vi "Flowmeter - revA.vi"() -> ()   [LabVIEW 2018]
doc: "This example demonstrates how to continuously perform period, frequency, pulse width, or two edge separation measurement types.\n\nThis example uses implicit timing, which means that a sample is acquired for every period of your input signal.\n\nFor instructions on how to connect your signals to the DAQ device, refer to your device documentation."
uses:
  <vilib>/Utility/error.llb/DialogType.ctl
  <vilib>/DAQmx/read.llb/DAQmx Read (Counter DBL 1Chan 1Samp).vi
  <vilib>/DAQmx/create/channels.llb/DAQmx Create Channel (CI-Frequency).vi
  <vilib>/DAQmx/configure/timing.llb/DAQmx Timing (Implicit).vi
  <vilib>/DAQmx/miscellaneous.llb/DAQmx Fill In Error Info.vi
  <resource>/objmgr/daqmx.rc
panel:
  out "K-Factor":dbl
  in  "K-Factor":dbl[](array[numeric])
  in  "Range":dbl[](array[numeric])
  out "GPM":dbl
  in  "counter":tag
  in  "CI.Freq.Term":tag
  out "Frequency":dbl
  in  "Stop":bool
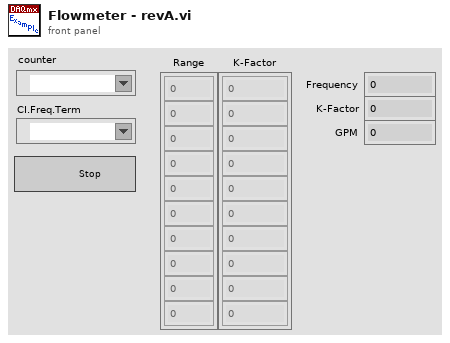
[diagram p1: front panel]
types:
  T1 = typedef "DialogType.ctl" = u16
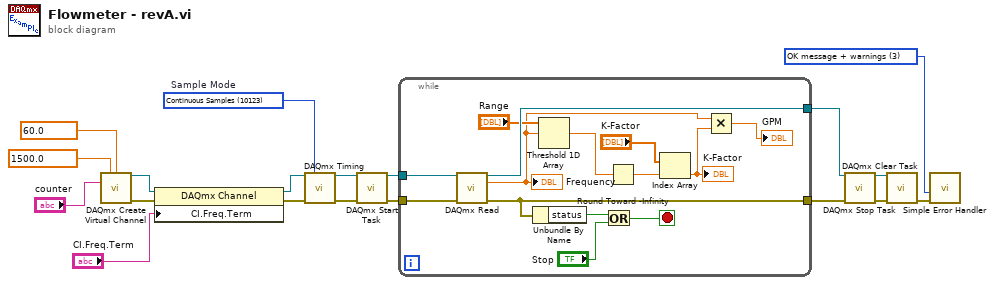
[diagram p0: block diagram]
diagram:
  w7 = T1 3 items=["no dialog", "OK message", "continue or stop message", "OK message + warnings", "continue/stop + warnings"] ("type of dialog (OK msg:1)")
  w19 = 10123 items=["Finite Samples"=10178, "Continuous Samples"=10123, "Hardware Timed Single Point"=12522]  # Sample Mode
  n1 = call-poly <vilib>:"DAQmx Create Virtual Channel.vi"("maximum value"=1500.0 ("Max Frequency"), "minimum value"=60.0 ("Min Frequency"), "counter"="counter") -> ("task out"=w6:refnum<k21>, "error out"=w5:errorcluster)  [unwired: 11 in]
  n2 = property class="DAQmx Channel"(reference=w6, error in=w5, "CI.Freq.Term"="CI.Freq.Term") -> (reference out=w17:refnum<k21>, error out=w18:errorcluster)
  n3 = call-poly <vilib>:"DAQmx Timing.vi"("task/channels in"=w17, "sample mode"=w19, "error in"=w18) -> ("task out"=w13:refnum<k21>, "error out"=w12:errorcluster)  [unwired: 11 in]
  n4 = call <vilib>:"DAQmx Start Task.vi"("task/channels in"=w13, "error in"=w12) -> ("task out"=w16:refnum<k21>, "error out"=w15:errorcluster)  [unwired: 12 in]
  n5 = while {
    tunnel: w16 -> [w33]
    tunnel: w15 -> [w32]
    tunnel: [w29] -> w8
    tunnel: [w30] -> w9
    stop <- w31 stop-if-true
    n6 = call-poly <vilib>:"DAQmx Read.vi"("task/channels in"=w33, "error in"=w32) -> ("task out"=w30:refnum<k21>, "data"=w20:dbl, "error out"=w29:errorcluster)  [unwired: 11 in]
    "Frequency" <- w20
    n7 = Unbundle By Name(w29) -> ("status"=w28:bool)
    n8 = Threshold 1D Array(2:w20, 3:"Range") -> (0:w24:dbl)  [unwired: 1 in]
    n9 = Or(x=w28, y="Stop") -> (x .or. y?=w31:bool)
    n10 = Round Toward -Infinity(1:w24) -> (0:w25:dbl)
    n11 = Index Array(array="K-Factor", index=w25) -> (element=w21:dbl)
    "K-Factor" <- w21
    n12 = Multiply(x=w20, y=w21) -> (x*y=→"GPM":dbl)
  }
  n13 = call <vilib>:"DAQmx Stop Task.vi"("task/channels in"=w9, "error in"=w8) -> ("task out"=w11:refnum<k21>, "error out"=w10:errorcluster)  [unwired: 12 in]
  n14 = call <vilib>:"DAQmx Clear Task.vi"("task in"=w11, "error in"=w10) -> ("error out"=w14:errorcluster)  [unwired: 13 in]
  n15 = call <vilib>:"Simple Error Handler.vi"("type of dialog (OK msg:1)"=w7, "error in (no error)"=w14) -> ()  [unwired: 3 in, 5 out]
